vi "PEXHDCAP60L2.vi"() -> ()   [LabVIEW 2020]
uses:
  <vilib>/userDefined/High Color/IMAQdx.ctl
  <vilib>/Utility/miscctls.llb/LVPointTypeDef.ctl
  LabVIEW 2020 Toolkits/toolkits_lv2020_32bit/Synchronization.llb/SynchRefs_SetGet.ctl
  LabVIEW 2020 Toolkits/VI Server Toolkit/VI Server Libraries/VI Server_SetControl.llb/VI Server_BOOL_Set.vi
  LabVIEW 2020 Toolkits/VI Server Toolkit/VI Server Libraries/VI Server_GetControl.llb/VI Server_STR_Get.vi
  LabVIEW 2020 Toolkits/VI Server Toolkit/VI Server Libraries/VI Server_Set Controls.llb/Set STR Control.vi
  LabVIEW 2020 Toolkits/VI Server Toolkit/VI Server Toolkit LV2013.lvlib
panel:
  in  "PASS":bool
  in  "DONE":bool
  in  "Manual.Open":bool caption="IDD.Open"
  in  "Help":bool
  in  "FP.Hide":bool caption="FrontPanel.Hide"
  out "System.Message":string caption="System Message"
  in  "EXIT":bool
  in  "Tab.Main":enum32{"Channel 1", "SETTINGS"}(tab)
  in  "Ch1.PartSerialNumber":string caption="Part Serial Number"
  in  "Ch1.SAVE":bool
  in  "Ch1.Image.Autosave":bool
  out "Ch1.AcquiredFrameRate":dbl caption="Frame Rate" format="%#_g f/sec"
  out "Ch1.AcquisitionTime":u32 caption="Acquisition Time"
  in  "Ch1.Acquire":bool
  in  "Ch1.NumberOfFrames":u32 caption="Number Of Frames"
  in  "Ch1.AcquisitionMode":u16(ring) caption="Acquisition Mode" items=["Single Frame", "Number of Frames", "Continious"]
  out "Ch1.Image":T1(plugin-control) caption="Image"
  out "Ch1.Image.Array":T1[](array[plugin-control]) caption="Image Array"
  in  "Ch1.ImagesFolder":path=path "C:/Program Files (x86)/Adobe/Acrobat Reader DC/Reader/AcroRd32.exe" caption="Images Folder"
  in  "Ch1.Camera":T2 caption="Ch1: Camera"
  in  "Setup.AdobeAcrobat.Path":path=path "C:/Program Files (x86)/Adobe/Acrobat Reader DC/Reader/AcroRd32.exe" caption="Acrobat Reader Path"
  in  "VI.WindowsTitle":string="PIXCI-SV7" caption="Windows Title"
  in  "UDP.Test.String2.Send":bool
  in  "UDP.Test.String2":string caption="UDP: Test String 2"
  in  "UDP.Port.BC":u16=58433 caption="UDP: Port.BC"
  in  "UDP.Port.RT":u16=58432 caption="UDP: Port.RT"
  in  "UDP.LocalPort.Write":u16=58434 caption="UDP: Local Port.Write"
  in  "UDP.IP.Address":string="234.5.6.7" caption="UDP: IP Address"
  in  "UDP.Test.String1.Send":bool
  in  "UDP.Test.String1":string caption="UDP: Test String 1"
  in  "UDP.Responce.String.Monitor":bool
  out "UDP.ExecEng.Message.String":string caption="UDP: Execution Engine Message String"
  out "error out":errorcluster
  in  "error in":errorcluster
  # "Build 0"
  # "Multicast IP addresses must be in the 224.0.0.0 to 239.255.255.255 range."
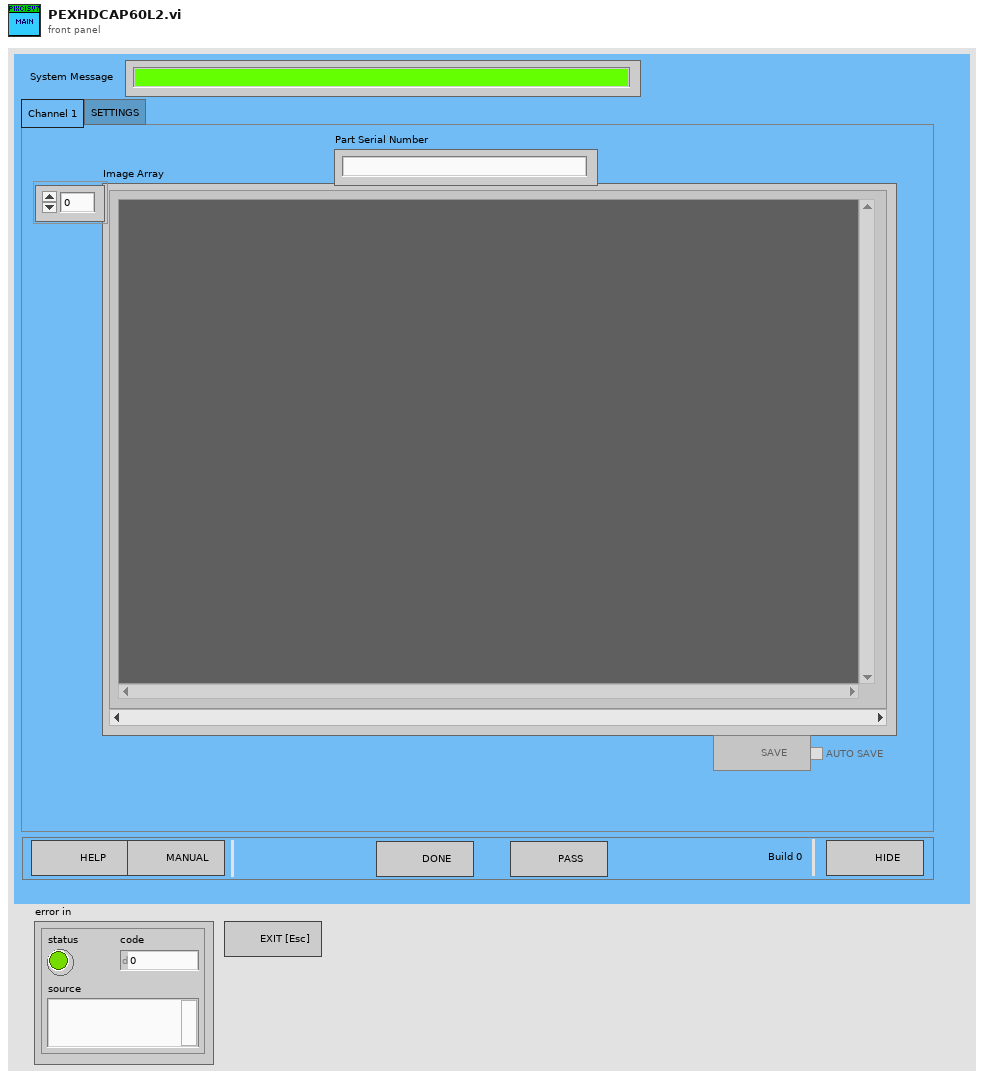
[diagram p1: front panel]
types:
  T1 = typedef "IMAQ Image.ctl" = refnum<image>
  T2 = typedef "IMAQdx.ctl" = refnum<k21>
  T3 = typedef "LVPointTypeDef.ctl" = cluster{"Horizontal":i16, "Vertical":i16}
  T4 = typedef "VI Server_RefsCluster.ctl" = cluster{"Labels":string[], "Refs":refnum<vi>[], "VI Ref":refnum<vi>}
  T5 = typedef "SynchRefs_SetGet.ctl" = enum16{"Set", "Get"}
  T6 = enum8{"Enabled", "Disabled", "Disabled and Grayed Out"}
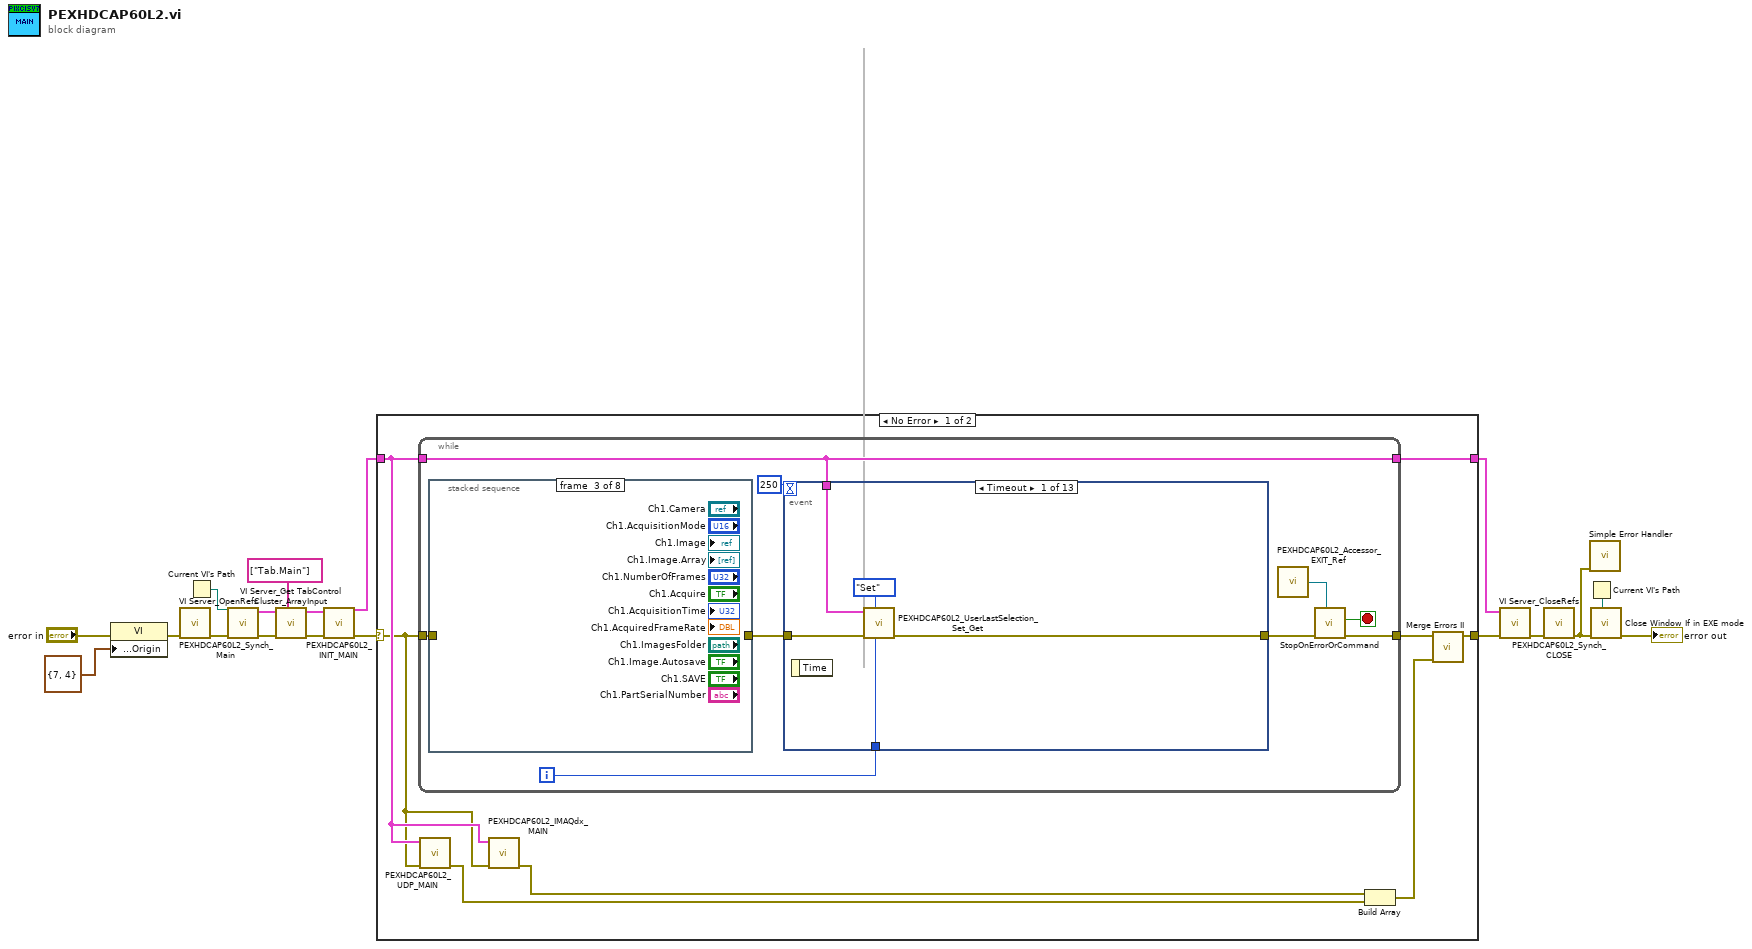
[diagram p0: block diagram]
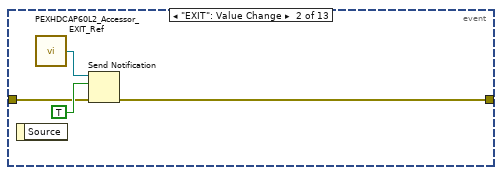
[diagram p2: hidden frame]
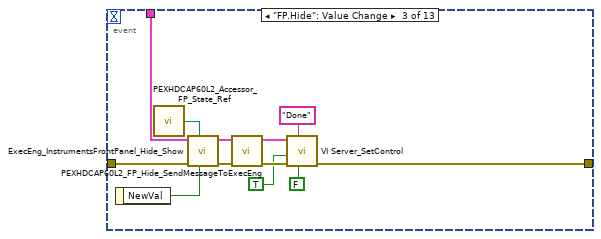
[diagram p3: hidden frame]
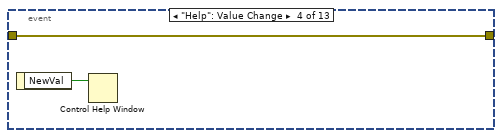
[diagram p4: hidden frame]
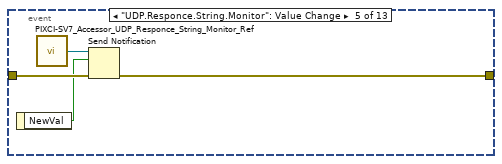
[diagram p5: hidden frame]
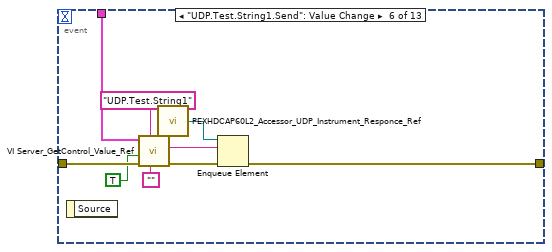
[diagram p6: hidden frame]
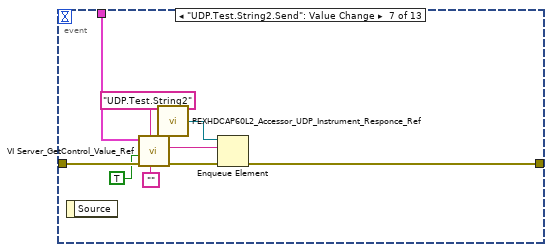
[diagram p7: hidden frame]
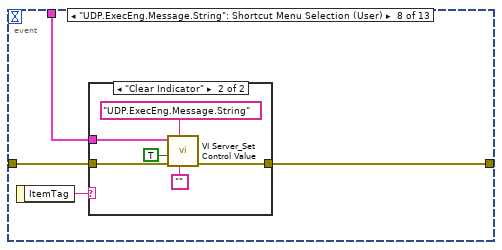
[diagram p8: hidden frame]
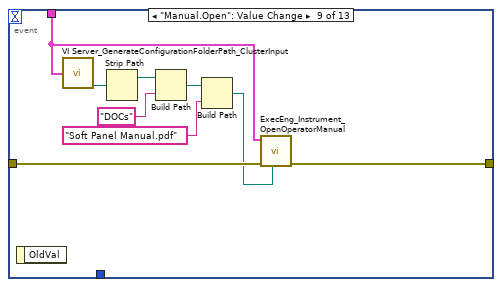
[diagram p10: hidden frame]
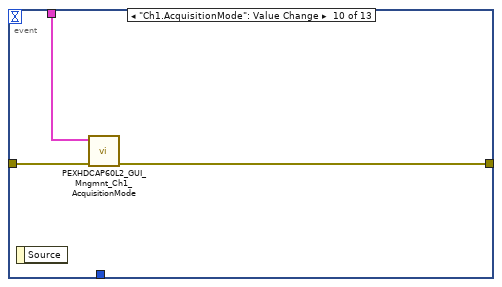
[diagram p11: hidden frame]
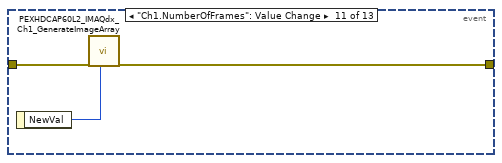
[diagram p12: hidden frame]
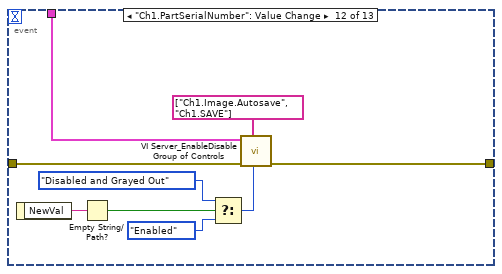
[diagram p13: hidden frame]
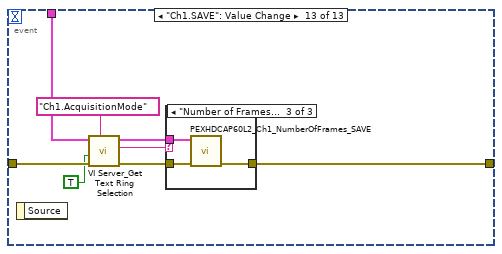
[diagram p14: hidden frame]
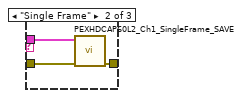
[diagram p16: hidden frame]
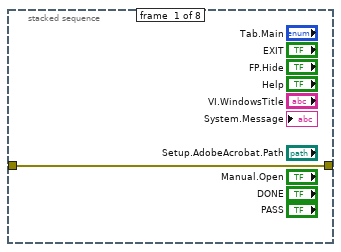
[diagram p17: hidden frame]
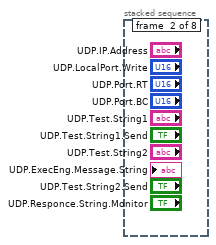
[diagram p18: hidden frame]
diagram:
  n1 = property class="VI"(error in="error in", "Front Panel Window:Origin"=T3 {"Horizontal"=7, "Vertical"=4}) -> (error out=w12:errorcluster)  [unwired: 1 in, 1 out]
  n2 = call "PEXHDCAP60L2_Synch_Main.vi"("error in"=w12) -> ("error out"=w13:errorcluster)  [unwired: 10 in]
  n3 = Current VI's Path() -> (path=w17:path)
  n4 = call "VI Server_OpenRefs.vi"("error in"=w13, "VI Path"=w17) -> ("error out"=w14:errorcluster, "VI Server.RefsCluster"=w15:T4)  [unwired: 8 in]
  n5 = call "VI Server_Get TabControl Cluster_ArrayInput.vi"("TabControl Labels[]"=string[] ["Tab.Main"], "error in"=w14, "VI Server Cluster"=w15) -> ("error out"=w11:errorcluster, "VI Server Cluster.OUT"=w10:T4)  [unwired: 7 in]
  n6 = call "PEXHDCAP60L2_INIT_MAIN.vi"("error in (no error)"=w11, "VI Server Cluster"=w10) -> ("error out"=w9:errorcluster, "VI Server Cluster DUP"=w8:T4)  [unwired: 8 in]
  n7 = case shown="No Error" w9 {
    selector: w9 -> [w20 w133]
    tunnel: [w23 w133] -> w2
    tunnel: w8 -> [w21 w132]
    tunnel: [w26 w132] -> w3
    frame No Error {
      n8 = while {
        tunnel: w20 -> [w35]
        tunnel: [w29] -> w24
        tunnel: w21 -> [w31]
        tunnel: [w31] -> w26
        i -> [w32]
        stop <- w28 stop-if-true
        n9 = stacked-sequence {
          tunnel: w35 -> [w131 _ _ _ _ _ _ _]
          tunnel: [w131 _ _ _ _ _ _ _] -> w34
          frame #0 {
          }
          frame #1 {
          }
          frame #2 {
          }
          frame #3 {
          }
          frame #4 {
          }
          frame #5 {
          }
          frame #6 {
          }
          frame #7 {
          }
        }
        n10 = event shown="[0] Timeout" {
          selector: _ -> [_ _ _ _ _ _ _ _ _ _ _ _ _]
          dyn-events: _ -> [_ _ _ _ _ _ _ _ _ _ _ _ _]
          timeout: 250 -> [_ _ _ _ _ _ _ _ _ _ _ _ _]
          tunnel: w34 -> [w39 w41 w56 w58 w62 w71 w80 w84 w99 w103 w106 w114 w123]
          tunnel: w32 -> [w38 _ _ _ _ _ _ _ _ _ _ _ _]
          tunnel: [w36 w43 w49 w58 w60 w69 w78 w82 w100 w101 w105 w113 w116] -> w30
          tunnel: w31 -> [w37 _ w53 _ _ w68 w77 w81 w98 w102 _ w112 w122]
          event Timeout {
            n11 = event-data() -> ()  [unwired: 1 in, 1 out]
            n12 = call "PEXHDCAP60L2_UserLastSelection_Set_Get.vi"("LoopCounter"=w38, "SynchRefs.Set/Get"=SynchRefs_SetGet."Set", "error in"=w39, "VI Server.RefsCluster"=w37) -> ("error out"=w36:errorcluster)  [unwired: 6 in, 1 out]
          }
          event "EXIT": Value Change {
            n13 = event-data() -> ()  [unwired: 1 in, 1 out]
            n14 = call "PEXHDCAP60L2_Accessor_EXIT_Ref.vi"() -> ("EXIT"=w44:refnum<notifier>)  [unwired: 6 in]
            n15 = Send Notification(notification=TRUE, notifier=w44, error in (no error)=w41) -> (error out=w43:errorcluster)  [unwired: 1 out]
          }
          event "FP.Hide": Value Change {
            n16 = event-data() -> ("NewVal"=w54:bool)  [unwired: 1 in]
            n17 = call "PEXHDCAP60L2_Accessor_FP_State_Ref.vi"() -> ("FP.State"=w51:refnum<notifier>)  [unwired: 6 in]
            n18 = call "ExecEng_InstrumentsFrontPanel_Hide_Show.vi"("FP.Hide/Show"=w54, "FP.State"=w51, "error in (no error)"=w56, "VI Server Cluster"=w53) -> ("error out"=w55:errorcluster, "VI Server Cluster DUP"=w52:T4)  [unwired: 6 in]
            n19 = call "PEXHDCAP60L2_FP_Hide_SendMessageToExecEng.vi"("error in (no error)"=w55, "VI Server Cluster"=w52) -> ("error out"=w50:errorcluster, "VI Server Cluster.DUP"=w48:T4)  [unwired: 8 in]
            n20 = call-poly "VI Server_SetControl.vi"("Data"=FALSE, "Control.Label"="Done", "error in"=w50, "SingleInstance"=TRUE, "VI Server.RefsCluster"=w48) -> ("error out"=w49:errorcluster)  [unwired: 4 in, 2 out]
          }
          event "Help": Value Change {
            n21 = event-data() -> ("NewVal"=w57:bool)  [unwired: 1 in]
            n22 = Control Help Window(1:w57) -> ()  [unwired: 1 in]
          }
          event "UDP.Responce.String.Monitor": Value Change {
            n23 = event-data() -> ("NewVal"=w59:bool)  [unwired: 1 in]
            n24 = call "PIXCI-SV7_Accessor_UDP_Responce_String_Monitor_Ref.vi"() -> ("UDP.ExecEng.Command.String.Monitor"=w61:refnum<notifier>)  [unwired: 6 in]
            n25 = Send Notification(notification=w59, notifier=w61, error in (no error)=w62) -> (error out=w60:errorcluster)  [unwired: 1 out]
          }
          event "UDP.Test.String1.Send": Value Change {
            n26 = event-data() -> ()  [unwired: 1 in, 1 out]
            n27 = call-poly "VI Server_GetControl_Value_Ref.vi"("DataType"="", "Control.Label"="UDP.Test.String1", "error in"=w71, "SingleInstance"=TRUE, "VI Server.RefsCluster"=w68) -> ("error out"=w70:errorcluster, "Value"=w63:string)  [unwired: 3 in, 2 out]
            n28 = call "PEXHDCAP60L2_Accessor_UDP_Instrument_Responce_Ref.vi"() -> ("UDP.Instrument.Responce.Q"=w64:refnum<queue>)  [unwired: 6 in]
            n29 = Enqueue Element(queue=w64, element=w63, error in (no error)=w70) -> (error out=w69:errorcluster)  [unwired: 1 in, 2 out]
          }
          event "UDP.Test.String2.Send": Value Change {
            n30 = event-data() -> ()  [unwired: 1 in, 1 out]
            n31 = call-poly "VI Server_GetControl_Value_Ref.vi"("DataType"="", "Control.Label"="UDP.Test.String2", "error in"=w80, "SingleInstance"=TRUE, "VI Server.RefsCluster"=w77) -> ("error out"=w79:errorcluster, "Value"=w72:string)  [unwired: 3 in, 2 out]
            n32 = call "PEXHDCAP60L2_Accessor_UDP_Instrument_Responce_Ref.vi"() -> ("UDP.Instrument.Responce.Q"=w73:refnum<queue>)  [unwired: 6 in]
            n33 = Enqueue Element(queue=w73, element=w72, error in (no error)=w79) -> (error out=w78:errorcluster)  [unwired: 1 in, 2 out]
          }
          event "UDP.ExecEng.Message.String": Shortcut Menu Selection (User) {
            n34 = event-data() -> ("ItemTag"=w83:string)  [unwired: 1 in]
            n35 = case shown="\"Clear Indicator\"" w83 {
              tunnel: w84 -> [w85 w91]
              tunnel: [w85 w90] -> w82
              tunnel: w81 -> [_ w89]
              frame "", Default {
              }
              frame "Clear Indicator" {
                n36 = call-poly "VI Server_Set Control Value.vi"("New Value"="", "Label"="UDP.ExecEng.Message.String" ("Control.Label"), "error in"=w91, "Single Instance (T)"=TRUE ("SingleInstance"), "VI Server Cluster"=w89) -> ("error out"=w90:errorcluster)  [unwired: 4 in, 2 out]
              }
            }
          }
          event "Manual.Open": Value Change {
            n37 = event-data() -> ()  [unwired: 1 in, 1 out]
            n38 = call "VI Server_GenerateConfigurationFolderPath_ClusterInput.vi"("VI Server Cluster"=w98) -> ("Configuration Folder Path"=w97:path)  [unwired: 11 in, 3 out]
            n39 = Strip Path(path=w97) -> (stripped path=w96:path)  [unwired: 1 out]
            n40 = Build Path(base path=w96, name or relative path="DOCs") -> (appended path=w94:path)
            n41 = Build Path(base path=w94, name or relative path="Soft Panel Manual.pdf") -> (appended path=w92:path)
            n42 = call "ExecEng_Instrument_OpenOperatorManual.vi"("Operations Manual Path"=w92, "error in"=w99, "VI Server.RefsCluster"=w98) -> ("error out"=w100:errorcluster)  [unwired: 8 in]
          }
          event "Ch1.AcquisitionMode": Value Change {
            n43 = event-data() -> ()  [unwired: 1 in, 1 out]
            n44 = call "PEXHDCAP60L2_GUI_Mngmnt_Ch1_AcquisitionMode.vi"("error in (no error)"=w103, "VI Server Cluster"=w102) -> ("error out"=w101:errorcluster)  [unwired: 9 in]
          }
          event "Ch1.NumberOfFrames": Value Change {
            n45 = event-data() -> ("NewVal"=w104:u32)  [unwired: 1 in]
            n46 = call "PEXHDCAP60L2_IMAQdx_Ch1_GenerateImageArray.vi"("Number Of Frames"=w104, "error in (no error)"=w106) -> ("error out"=w105:errorcluster)  [unwired: 9 in]
          }
          event "Ch1.PartSerialNumber": Value Change {
            n47 = event-data() -> ("NewVal"=w111:string)  [unwired: 1 in]
            n48 = Empty String/Path?(string/path=w111) -> (empty?=w110:bool)
            n49 = Select(t=T6."Disabled and Grayed Out" ("Enable/Disable"), s=w110, f=T6."Enabled") -> (s? t:f=w107:T6)
            n50 = call "VI Server_EnableDisable Group of Controls.vi"("Enable/Disable"=w107, "Labels.Array"=string[] ["Ch1.Image.Autosave", "Ch1.SAVE"], "error in"=w114, "VI Server Cluster"=w112) -> ("error out"=w113:errorcluster)  [unwired: 5 in, 2 out]
          }
          event "Ch1.SAVE": Value Change {
            n51 = event-data() -> ()  [unwired: 1 in, 1 out]
            n52 = call "VI Server_Get Text Ring Selection.vi"("Label"="Ch1.AcquisitionMode", "error in"=w123, "Single Instance (T)"=TRUE, "VI Server Cluster"=w122) -> ("error out"=w119:errorcluster, "Selection"=w118:string, "VI Server Custer.DUP"=w117:T4)  [unwired: 2 in, 3 out]
            n53 = case shown="\"Number of Frames\"" w118 {
              tunnel: w119 -> [w124 w127 w130]
              tunnel: w117 -> [_ w126 w129]
              tunnel: [w124 w125 w128] -> w116
              frame "False", Default {
              }
              frame "Single Frame" {
                n54 = call "PEXHDCAP60L2_Ch1_SingleFrame_SAVE.vi"("error in (no error)"=w127, "VI Server Cluster"=w126) -> ("error out"=w125:errorcluster)  [unwired: 8 in, 1 out]
              }
              frame "Number of Frames" {
                n55 = call "PEXHDCAP60L2_Ch1_NumberOfFrames_SAVE.vi"("error in (no error)"=w130, "VI Server Cluster"=w129) -> ("error out"=w128:errorcluster)  [unwired: 8 in, 1 out]
              }
            }
          }
        }
        n56 = call "PEXHDCAP60L2_Accessor_EXIT_Ref.vi"() -> ("EXIT"=w27:refnum<notifier>)  [unwired: 6 in]
        n57 = call "StopOnErrorOrCommand.vi"("STOP"=w27, "error in (no error)"=w30) -> ("error out"=w29:errorcluster, "STOP"=w28:bool)  [unwired: 8 in]
      }
      n58 = call "PEXHDCAP60L2_UDP_MAIN.vi"("error in (no error)"=w20, "VI Server.RefsCluster"=w21) -> ("error out"=w25:errorcluster)  [unwired: 9 in]
      n59 = call "PEXHDCAP60L2_IMAQdx_MAIN.vi"("error in (no error)"=w20, "VI Server.RefsCluster"=w21) -> ("error out"=w19:errorcluster)  [unwired: 9 in]
      n60 = Build Array(w19, w25) -> (w22:errorcluster[])
      n61 = call "Merge Errors II.vi"("error array in"=w22, "error in 1 (no error)"=w24) -> ("error out.DUP"=w23:errorcluster)  [unwired: 4 in, 1 out]
    }
    frame Error {
    }
  }
  n62 = call "VI Server_CloseRefs.vi"("error in"=w2, "VI Server.RefsCluster"=w3) -> ("error out"=w7:errorcluster)  [unwired: 9 in]
  n63 = call "PEXHDCAP60L2_Synch_CLOSE.vi"("error in"=w7) -> ("error out"=w1:errorcluster)  [unwired: 10 in]
  n64 = Current VI's Path() -> (path=w5:path)
  n65 = call <vilib>:"Simple Error Handler.vi"("error in (no error)"=w1) -> ()  [unwired: 4 in, 5 out]
  n66 = call "Close Window If in EXE mode.vi"("TopLevelVI Path"=w5, "error in"=w1) -> ("error out"=→"error out":errorcluster)  [unwired: 9 in]
